vi "CT_GFDIGtoGraph.vi"(8 "GFDIG Graph Plots":string[][](array[string]), 10 "GFDIG Waveforms":waveform(dbl)[](array[waveform])=[{"t0"=timestamp(3355420112.226375 s since 1904-01-01), "dt"=5e-08, "Y"=array[59968 elements], "attributes"=variant("NI_ChannelName"=variant(string "PVD1"))}, {"t0"=timestamp(3355420112.226375 s since 1904-01-01), "dt"=5e-08, "Y"=array[59968 elements], "attributes"=variant("NI_ChannelName"=variant(string "PVD2"))}, {"t0"=timestamp(3355420112.226375 s since 1904-01-01), "dt"=5e-08, "Y"=array[59968 elements], "attributes"=variant("NI_ChannelName"=variant(string "PVD3\nPVD3"))}, {"t0"=timestamp(3355420112.226375 s since 1904-01-01), "dt"=5e-08, "Y"=array[59968 elements], "attributes"=variant("NI_ChannelName"=variant(string "PVD4"))}, {"t0"=timestamp(3355420112.226375 s since 1904-01-01), "dt"=5e-08, "Y"=array[59968 elements], "attributes"=variant("NI_ChannelName"=variant(string "PVD5"))}, {"t0"=timestamp(3355420112.226375 s since 1904-01-01), "dt"=5e-08, "Y"=array[59968 elements], "attributes"=variant("NI_ChannelName"=variant(string "PVD6"))}, {"t0"=timestamp(3355420112.226375 s since 1904-01-01), "dt"=5e-08, "Y"=array[59968 elements], "attributes"=variant("NI_ChannelName"=variant(string "PVD8"))}, {"t0"=timestamp(3355420112.226375 s since 1904-01-01), "dt"=5e-08, "Y"=array[59968 elements], "attributes"=variant("NI_ChannelName"=variant(string "PVD10"))}, {"t0"=timestamp(3355420112.226375 s since 1904-01-01), "dt"=5e-08, "Y"=array[59968 elements], "attributes"=variant("NI_ChannelName"=variant(string "PVD11"))}, {"t0"=timestamp(3355420112.226375 s since 1904-01-01), "dt"=5e-08, "Y"=array[59968 elements], "attributes"=variant("NI_ChannelName"=variant(string "PVD12"))}]) -> (2 "Graph Array":waveform(dbl)[][](array[waveform])=[[{"t0"=timestamp(3355420112.226375 s since 1904-01-01), "dt"=5e-08, "Y"=array[59968 elements], "attributes"=variant("NI_ChannelName"=variant(string "PVD1"))}, {"t0"=timestamp(3355420112.226375 s since 1904-01-01), "dt"=5e-08, "Y"=array[59968 elements], "attributes"=variant("NI_ChannelName"=variant(string "PVD2"))}, {"t0"=timestamp(3355420112.226375 s since 1904-01-01), "dt"=5e-08, "Y"=array[59968 elements], "attributes"=variant("NI_ChannelName"=variant(string "PVD4"))}, {"t0"=timestamp(3355420112.226375 s since 1904-01-01), "dt"=5e-08, "Y"=array[59968 elements], "attributes"=variant("NI_ChannelName"=variant(string "PVD5"))}, {"t0"=timestamp(3355420112.226375 s since 1904-01-01), "dt"=5e-08, "Y"=array[59968 elements], "attributes"=variant("NI_ChannelName"=variant(string "PVD6"))}, {"t0"=timestamp(3355420112.226375 s since 1904-01-01), "dt"=5e-08, "Y"=array[59968 elements], "attributes"=variant("NI_ChannelName"=variant(string "PVD8"))}, {"t0"=timestamp(3355420112.226375 s since 1904-01-01), "dt"=5e-08, "Y"=array[59968 elements], "attributes"=variant("NI_ChannelName"=variant(string "PVD10"))}, {"t0"=timestamp(3355420112.226375 s since 1904-01-01), "dt"=5e-08, "Y"=array[59968 elements], "attributes"=variant("NI_ChannelName"=variant(string "PVD11"))}, {"t0"=timestamp(3355420112.226375 s since 1904-01-01), "dt"=5e-08, "Y"=array[59968 elements], "attributes"=variant("NI_ChannelName"=variant(string "PVD12"))}], [{"t0"=timestamp(0 s since 1904-01-01), "dt"=1.0, "Y"=[]}, {"t0"=timestamp(0 s since 1904-01-01), "dt"=1.0, "Y"=[]}, {"t0"=timestamp(0 s since 1904-01-01), "dt"=1.0, "Y"=[]}, {"t0"=timestamp(0 s since 1904-01-01), "dt"=1.0, "Y"=[]}, {"t0"=timestamp(0 s since 1904-01-01), "dt"=1.0, "Y"=[]}, {"t0"=timestamp(0 s since 1904-01-01), "dt"=1.0, "Y"=[]}, {"t0"=timestamp(0 s since 1904-01-01), "dt"=1.0, "Y"=[]}, {"t0"=timestamp(0 s since 1904-01-01), "dt"=1.0, "Y"=[]}, {"t0"=timestamp(0 s since 1904-01-01), "dt"=1.0, "Y"=[]}], [{"t0"=timestamp(0 s since 1904-01-01), "dt"=1.0, "Y"=[]}, {"t0"=timestamp(0 s since 1904-01-01), "dt"=1.0, "Y"=[]}, {"t0"=timestamp(0 s since 1904-01-01), "dt"=1.0, "Y"=[]}, {"t0"=timestamp(0 s since 1904-01-01), "dt"=1.0, "Y"=[]}, {"t0"=timestamp(0 s since 1904-01-01), "dt"=1.0, "Y"=[]}, {"t0"=timestamp(0 s since 1904-01-01), "dt"=1.0, "Y"=[]}, {"t0"=timestamp(0 s since 1904-01-01), "dt"=1.0, "Y"=[]}, {"t0"=timestamp(0 s since 1904-01-01), "dt"=1.0, "Y"=[]}, {"t0"=timestamp(0 s since 1904-01-01), "dt"=1.0, "Y"=[]}]])   [LabVIEW 2009]
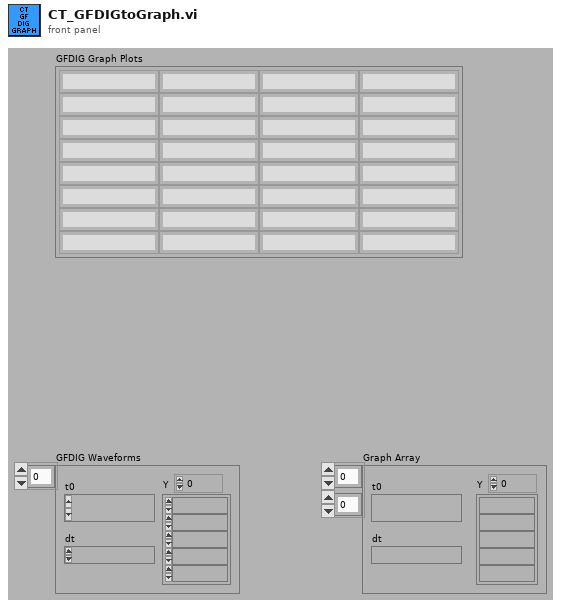
[diagram p1: front panel]
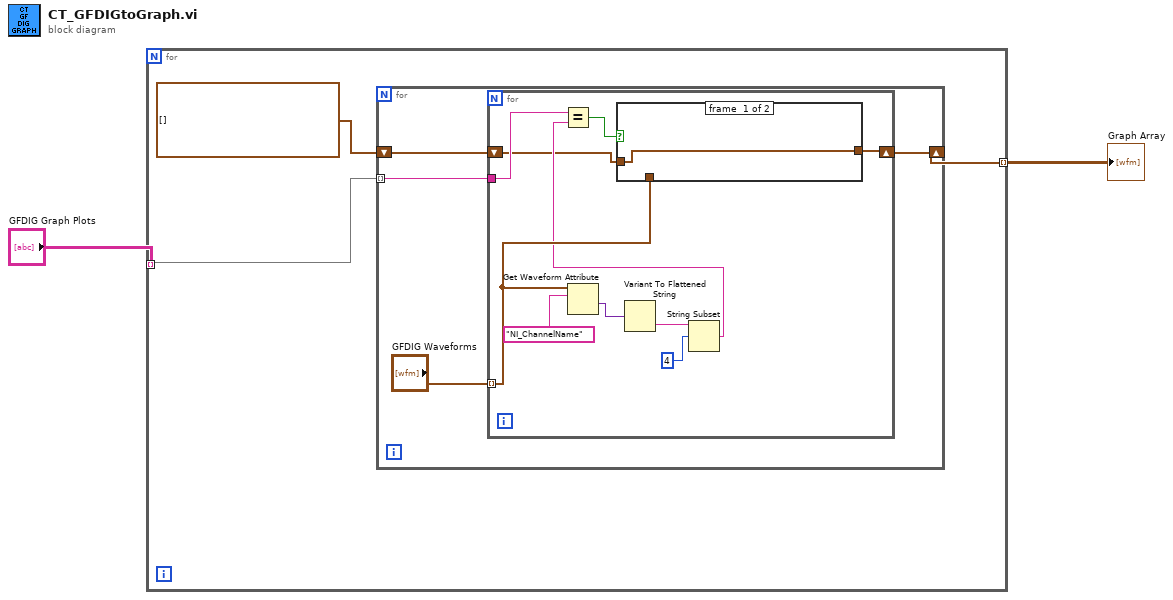
[diagram p0: block diagram]
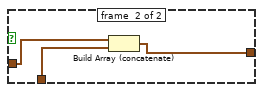
[diagram p2: hidden frame]
diagram:
  n1 = for {
    tunnel: "GFDIG Graph Plots" -> [w5] mode=indexing
    tunnel: [w3] -> w1 mode=indexing
    n2 = for {
      shift-right: [w7] -> w3
      shift-left: waveform(dbl)[] [] -> [w6]
      tunnel: w5 -> [w9] mode=indexing
      n3 = for {
        tunnel: w9 -> [w18]
        tunnel: "GFDIG Waveforms" -> [w13] mode=indexing
        shift-right: [w11] -> w7
        shift-left: w6 -> [w10]
        n4 = Get Waveform Attribute(6:"NI_ChannelName", 7:w13) -> (1:w15:variant)  [unwired: 2 in, 3 out]
        n5 = Variant To Flattened String(Variant=w15) -> (data string=w16:string)  [unwired: 1 out]
        n6 = String Subset(string=w16, offset (0)=4) -> (substring=w12:string)  [unwired: 1 in]
        n7 = Equal?(x=w18, y=w12) -> (x = y?=w19:bool)
        n8 = case shown="True" w19 {
          tunnel: [w20 w23] -> w11
          tunnel: w10 -> [w20 w22]
          tunnel: w13 -> [_ w21]
          frame #0 {
          }
          frame #1 {
            n9 = Build Array (concatenate)(w22, w21) -> (w23:waveform(dbl)[])
          }
        }
      }
    }
  }
  "Graph Array" <- w1
